vi "PRODUCT_COUNT_DOWNLOAD.vi"(8 "error in (no error)":errorcluster, 9 "Quantity Day":i32[][](array[numeric]), 10 "appended array":refnum<vi>[](array[refnum])) -> (0 "error out":errorcluster)   [LabVIEW 2017]
panel:
  in  "Quantity PER DAYS":i32
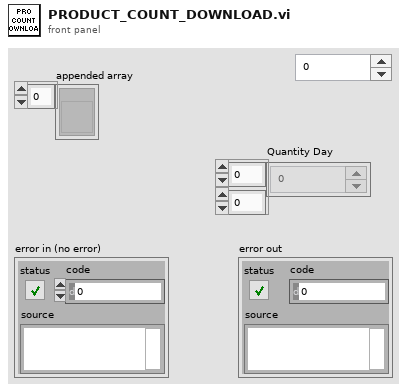
[diagram p1: front panel]
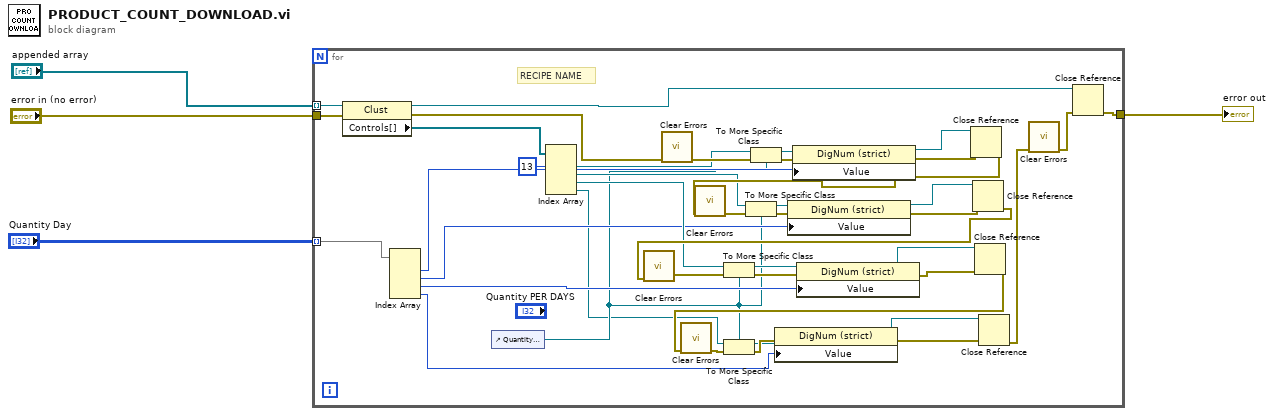
[diagram p0: block diagram]
diagram:
  n1 = for {
    tunnel: [w43] -> w2
    tunnel: "appended array" -> [w46] mode=indexing
    tunnel: "error in (no error)" -> [w45]
    tunnel: "Quantity Day" -> [w11] mode=indexing
    # "RECIPE NAME"
    n2 = property class="Clust"(reference=w46, error in=w45) -> (reference out=w42:refnum<vi>, error out=w44:errorcluster, "Controls[]"=w40:refnum<vi>[])
    n3 = Index Array(array=w11) -> (element #1=w29:i32, element #2=w14:i32, element #3=w13:i32, element #4=w12:i32)  [unwired: 4 in]
    n4 = control-ref of="Quantity PER DAYS"() -> (w6:refnum<vi>)
    n5 = Index Array(array=w40, index #1=13 ("index")) -> (element #1=w15:refnum<vi>, element #2=w19:refnum<vi>, element #3=w24:refnum<vi>, element #4=w5:refnum<vi>)  [unwired: 3 in]
    n6 = call <vilib>:"Clear Errors.vi"("error in (no error)"=w44) -> ("error out"=w18:errorcluster)  [unwired: 5 in, 1 out]
    n7 = To More Specific Class(target class=w6, reference=w15, error in=w18) -> (specific class reference=w16:refnum<vi>, error out=w17:errorcluster)
    n8 = property class="DigNum (strict)"(reference=w16, error in=w17, "Value"=w29) -> (reference out=w33:refnum<vi>, error out=w41:errorcluster)
    n9 = Close Reference(reference=w33, error in (no error)=w41) -> (error out=w36:errorcluster)
    n10 = call <vilib>:"Clear Errors.vi"("error in (no error)"=w36) -> ("error out"=w22:errorcluster)  [unwired: 5 in, 1 out]
    n11 = To More Specific Class(target class=w6, reference=w19, error in=w22) -> (specific class reference=w20:refnum<vi>, error out=w21:errorcluster)
    n12 = property class="DigNum (strict)"(reference=w20, error in=w21, "Value"=w14) -> (reference out=w32:refnum<vi>, error out=w38:errorcluster)
    n13 = Close Reference(reference=w32, error in (no error)=w38) -> (error out=w35:errorcluster)
    n14 = call <vilib>:"Clear Errors.vi"("error in (no error)"=w35) -> ("error out"=w25:errorcluster)  [unwired: 5 in, 1 out]
    n15 = To More Specific Class(target class=w6, reference=w24, error in=w25) -> (specific class reference=w23:refnum<vi>, error out=w26:errorcluster)
    n16 = property class="DigNum (strict)"(reference=w23, error in=w26, "Value"=w13) -> (reference out=w31:refnum<vi>, error out=w37:errorcluster)
    n17 = Close Reference(reference=w31, error in (no error)=w37) -> (error out=w34:errorcluster)
    n18 = call <vilib>:"Clear Errors.vi"("error in (no error)"=w34) -> ("error out"=w28:errorcluster)  [unwired: 5 in, 1 out]
    n19 = To More Specific Class(target class=w6, reference=w5, error in=w28) -> (specific class reference=w10:refnum<vi>, error out=w27:errorcluster)
    n20 = property on="Property Node" class="DigNum (strict)"(reference=w10, error in=w27, "Value"=w12) -> (reference out=w30:refnum<vi>, error out=w7:errorcluster)
    n21 = Close Reference(reference=w30, error in (no error)=w7) -> (error out=w9:errorcluster)
    n22 = call <vilib>:"Clear Errors.vi"("error in (no error)"=w9) -> ("error out"=w8:errorcluster)  [unwired: 5 in, 1 out]
    n23 = Close Reference(reference=w42, error in (no error)=w8) -> (error out=w43:errorcluster)
  }
  "error out" <- w2
